vi "Get_RegData_TypeString.vi"(8 "error in (no error)":errorcluster, 11 "RegData_String in":refnum<class "IB_RegData_String.lvclass">) -> (0 "error out":errorcluster, 2 "Type String":string, 3 "RegData_String out":refnum<class "IB_RegData_String.lvclass">)   [LabVIEW 2020, in "IB_RegData_String.lvclass"]
uses:
  <vilib>/AppBuilder/IB_Classes/RegData/RegData_String/IB_RegData_String.lvclass
  <vilib>/AppBuilder/IB_Classes/RegData/RegData_String/IB_RegData_String.lvclass/IB_RegData_String.ctl
  <resource>/Framework/Providers/Builds/Installer/CDK_GLOBAL_STRINGS.vi
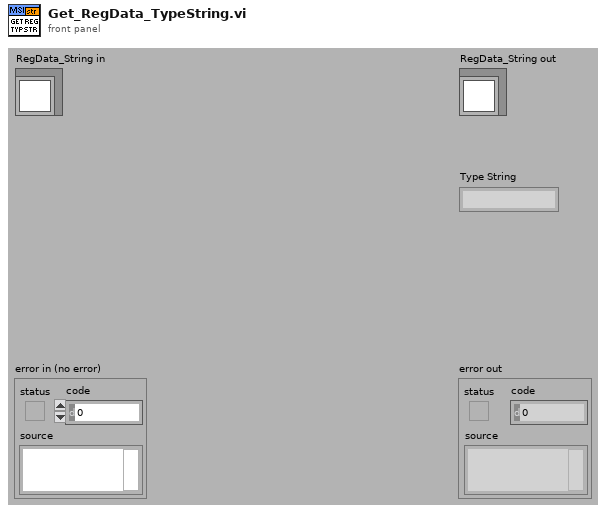
[diagram p1: front panel]
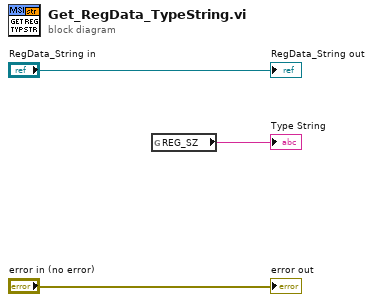
[diagram p0: block diagram]
diagram:
  n1 = global read "CDK_GLOBAL_STRINGS.vi" "REG_SZ"() -> (→"Type String":string)
  "error out" <- "error in (no error)"
  "RegData_String out" <- "RegData_String in"
